vi "SONG.vi"() -> ()   [LabVIEW 2016]
panel:
  out "SONG":string
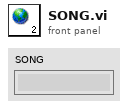
[diagram p1: front panel]
diagram:
